vi "Initial position.vi"(8 "error in (no error)":errorcluster, 11 "Scanner in":refnum<class "Scanner.lvclass">) -> (0 "error out":errorcluster, 2 "Initial positions":dbl[](array[numeric]), 3 "Scanner out":refnum<class "Scanner.lvclass">)   [LabVIEW 2017, in "Scanner.lvclass"]
uses:
  Scanner.lvclass
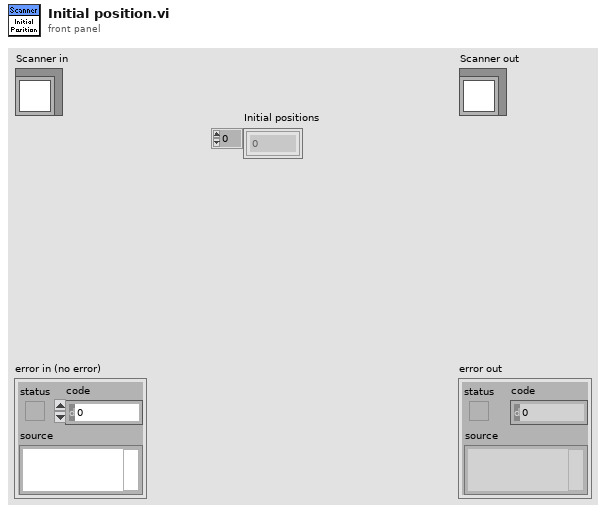
[diagram p1: front panel]
types:
  T1 = typedef "Scanner.lvclass/Range.ctl" = cluster{"xi":dbl, "xf":dbl, "dx":dbl, "Return to...?":bool, "Return to":dbl}
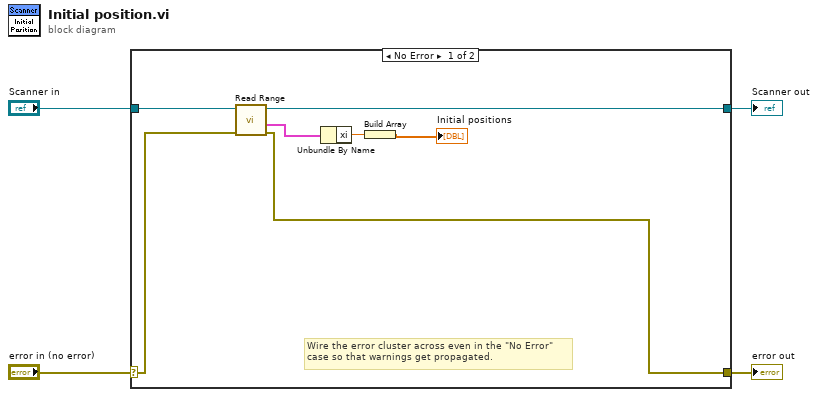
[diagram p0: block diagram]
diagram:
  n1 = case shown="No Error" "error in (no error)" {
    selector: "error in (no error)" -> [w6 w13]
    tunnel: [w5 w13] -> w3
    tunnel: [w9 w12] -> w1
    tunnel: "Scanner in" -> [w10 w12]
    frame No Error {
      # "Wire the error cluster across even in the \"No Error\"\ncase so that warnings get propagated."
      n2 = call-dynamic "Read Range.vi"("error in (no error)"=w6, "Scanner.lvclass in"=w10) -> ("error out"=w5:errorcluster, "Range"=w11:T1, "Scanner.lvclass out"=w9:refnum<class "Scanner.lvclass">)  [unwired: 7 out]
      n3 = Unbundle By Name(w11) -> ("xi"=w8:dbl)
      n4 = Build Array(w8) -> (→"Initial positions":dbl[])
    }
    frame Error {
    }
  }
  "error out" <- w3
  "Scanner out" <- w1
